vi "bounceball.vi"() -> ()   [LabVIEW 2017]
panel:
  in  "initial velocity":dbl
  in  "Bouncing constant":dbl
  out "Waveform Chart":dbl(graph)
  out "height":dbl(slide) scale=0.0..150.0
  in  "stop":bool
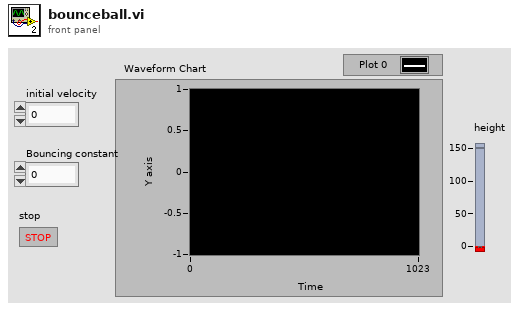
[diagram p1: front panel]
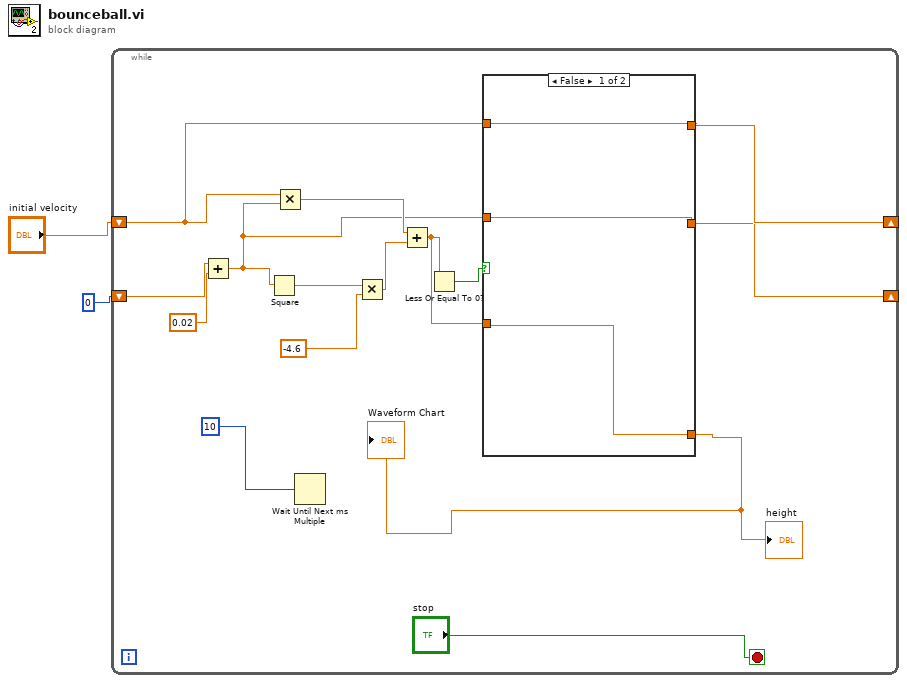
[diagram p0: block diagram]
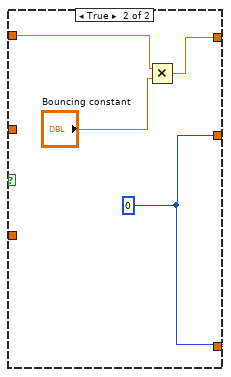
[diagram p2: hidden frame]
diagram:
  n1 = while {
    shift-right: [w6] -> _
    shift-left: 0 -> [w17]
    shift-right: [w7] -> _
    shift-left: "initial velocity" -> [w8]
    stop <- "stop" stop-if-true
    n2 = Add(x=w17, y=0.02) -> (x+y=w10:dbl)
    n3 = Square(x=w10) -> (x^2=w15:dbl)
    n4 = Multiply(x=w8, y=w10) -> (x*y=w13:dbl)
    n5 = Wait Until Next ms Multiple(millisecond multiple=10) -> ()  [unwired: 1 out]
    n6 = Multiply(x=w15, y=-4.6) -> (x*y=w12:dbl)
    n7 = Add(x=w13, y=w12) -> (x+y=w9:dbl)
    n8 = Less Or Equal To 0?(x=w9) -> (x <= 0?=w11:bool)
    n9 = case shown="False" w11 {
      tunnel: w10 -> [w20 _]
      tunnel: w9 -> [w18 _]
      tunnel: w8 -> [w19 w24]
      tunnel: [w19 w23] -> w7
      tunnel: [w20 w22] -> w6
      tunnel: [w18 w22] -> w3
      frame False {
      }
      frame True {
        w22 = 0
        n10 = Multiply(x=w24, y="Bouncing constant") -> (x*y=w23:dbl)
      }
    }
    "height" <- w3
    "Waveform Chart" <- w3
  }
